vi "Process-Logging.vi"(9 "Wait on post-processing":refnum<k4>, 10 "Queues Cluster":T1, 11 "Data-gen queue":T2) -> (0 "error out":errorcluster)   [LabVIEW 2020]
uses:
  Logging/Typedefs/ROI File Generator Queue Ref.ctl
  Typedefs/Logging queue element.ctl
  Typedefs/Imaging Protocols enum.ctl
  Typedefs/Frame Size.ctl
  Typedefs/Acquired points count.ctl
  User Interface/Queue/Message Queue/Typedefs/All Message Queues.ctl
  User Interface/Queue/Message Queue/Typedefs/Message Cluster.ctl
  Global Variables/General Globals.vi
panel:
  out "Loop iterations":i32
  out "Number of trials closed":u32
  out "Loop period (ms)":u32
  # "TIME-CRITICAL MODULE"
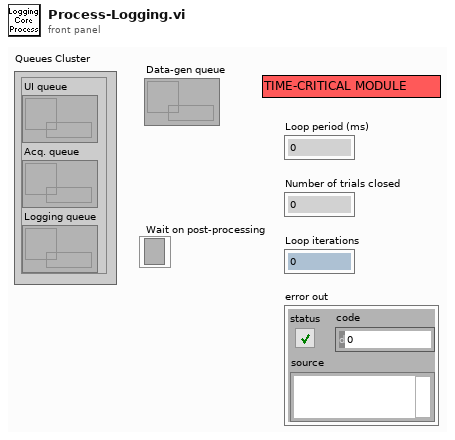
[diagram p1: front panel]
types:
  T1 = typedef "All Message Queues.ctl" = cluster{"UI queue":refnum<queue>, "Acq. queue":refnum<queue>, "Logging queue":refnum<queue>}
  T2 = typedef "ROI File Generator Queue Ref.ctl" = refnum<queue>
  T3 = cluster{"TDMS group name":string, "TDMS channel names array":string[]}
  T4 = typedef "Live graph data queue ref.ctl" = refnum<queue>
  T5 = typedef "Live imaging queue element.ctl" = cluster{"Red channel":T6, "Green channel":T6, "Ref Red channel":T6, "Ref Green channel":T6, "Mov cor":bool}
  T6 = typedef "IMAQ Image.ctl" = refnum<image>
  T7 = typedef "Logging queue element.ctl" = cluster{"Imaging Protocol":T8, "Number of Trials":u16, "Frame Size":T9, "# Averaged frames":u16, "Dwell time (us)":dbl, "Index of Z-plane":i32, "Timelapse?":bool, "Logging process is active":bool, "Speed logging enabled":bool, "tdms file ref":refnum<k34>, "path":path, "Trial Number":i32, "Expected # points acquired":bool, "Manually stopped":bool, "Last trial":bool, "Ch0 data":u32[], "Ch1 data":u32[], "Ref Data":u32[], "Ref Frame Time":u64[], "Image Time":u64[], "Continuous Time":u64[], "Ref X Length":u16, "Ref Y Length":u16, "# Ref Averaged frames":u16, "Ref Dwell time (us)":dbl, "Points acquired":T10, "HW Timings File":refnum<file>}
  T8 = typedef "Imaging Protocols enum.ctl" = enum16{"AOL Z-Stack", "Motor Z Stack", "Functional Acquisition", "Single Plane Acquisition", "Volume Acquisition", "Live Imaging", "Live Plane Imaging", "Live Volume Imaging"}
  T9 = typedef "Frame Size.ctl" = u16
  T10 = typedef "Acquired points count.ctl" = cluster{"Ch0 last trial":u64, "Ch1 last trial":u64, "All trials":u64}
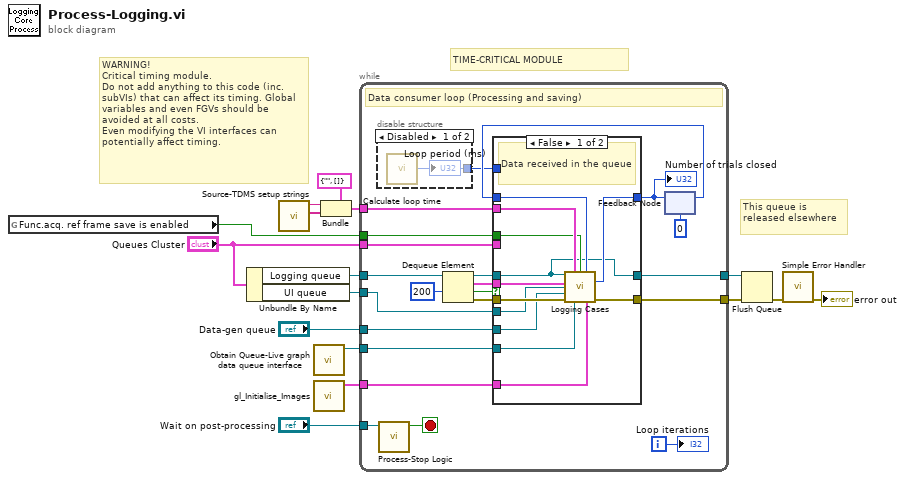
[diagram p0: block diagram]
diagram:
  # "WARNING!\nCritical timing module.\nDo not add anything to this code (inc. subVIs) that can affect its timing. Global variables and even FGVs should be avoided at all costs.\nEven modifying the VI interfaces can potentially affect timing."
  # "TIME-CRITICAL MODULE"
  # "This queue is released elsewhere"
  n1 = global read "General Globals.vi" "Func.acq. ref frame save is enabled"() -> (w2:bool)
  n2 = Unbundle By Name("Queues Cluster") -> ("Logging queue"=w4:refnum<queue>, "UI queue"=w1:refnum<queue>)
  n3 = call "Source-TDMS setup strings.vi"() -> ("Functional imaging TDMS channel names array"=w6:string[], "TDMS group name"=w7:string)  [unwired: 10 in]
  n4 = call "Obtain Queue-Live graph data queue interface.vi"() -> ("Live graphs queue"=w14:T4)  [unwired: 10 in, 1 out]
  n5 = call "gl_Initialise_Images.vi"() -> ("Live image refs"=w13:T5)  [unwired: 11 in]
  n6 = Bundle(cluster=T3 {"TDMS group name"="", "TDMS channel names array"=[]} ("Channel info"), "TDMS group name"=w7, "TDMS channel names array"=w6) -> (w5:T3)
  n7 = while {
    tunnel: [w35] -> w9
    tunnel: "Data-gen queue" -> [w33]
    tunnel: w13 -> [w31]
    tunnel: w14 -> [w29]
    tunnel: w4 -> [w34]
    tunnel: [w21] -> w10
    tunnel: "Wait on post-processing" -> [w22]
    tunnel: w5 -> [w24]
    tunnel: "Queues Cluster" -> [w20]
    tunnel: w2 -> [w19]
    tunnel: w1 -> [w18]
    i -> [w30]
    stop <- w23 stop-if-true
    # "Data consumer loop (Processing and saving)"
    n8 = disable-structure shown="Disabled" {
      disable-tunnel: [w39 _] -> w25
      frame Disabled {
        n9 = call <userlib>:"Calculate loop time.vi"() -> ("Loop time (ms)"=w39:u32)  [unwired: 11 in]
        "Loop period (ms)" <- w39
      }
      frame Enabled {
      }
    }
    n10 = call "Process-Stop Logic.vi"("Wait on post-processing"=w22) -> ("Abort logging"=w23:bool)  [unwired: 10 in]
    n11 = Dequeue Element(queue=w34, timeout in ms (-1)=200) -> (queue out=w17:refnum<queue>, element=w37:T7, timed out?=w28:bool, error out=w38:errorcluster)  [unwired: 1 in]
    n12 = feedback #1(u32 0 ("Number of files closed")) -> (w32:u32)
    n13 = case shown="False" w28 {
      tunnel: [w51 w54] -> w35
      tunnel: w38 -> [w50 w54]
      tunnel: w37 -> [w48 _]
      tunnel: w33 -> [w49 _]
      tunnel: [w43 w53] -> w27
      tunnel: w32 -> [w44 w53]
      tunnel: w31 -> [w46 _]
      tunnel: w29 -> [w47 _]
      tunnel: w17 -> [w41 w52]
      tunnel: w25 -> [_ _]
      tunnel: w24 -> [w45 _]
      tunnel: [w41 w52] -> w21
      tunnel: w20 -> [_ _]
      tunnel: w19 -> [w42 _]
      tunnel: w18 -> [w40 _]
      frame False {
        # "Data received in the queue"
        n14 = call "Logging Cases.vi"("Logging queue"=w41, "Channel info"=w45, "Enable ref saving during functional acq."=w42, "Number of files closed in"=w44, "Logging queue element in"=w48, "UI queue"=w40, "Data-gen queue"=w49, "error in"=w50, "Live graph data queue in"=w47, "Image array"=w46) -> ("Number of TDMS files closed"=w43:u32, "error out"=w51:errorcluster)  [unwired: 4 in]
      }
      frame True {
        # "Timed out (200ms). This case allows stopping the loop correctly."
      }
    }
    "Number of trials closed" <- w27
    n15 = feedback-in #1(w27) -> ()
    "Loop iterations" <- w30
  }
  n16 = Flush Queue(queue=w10, error in (no error)=w9) -> (error out=w11:errorcluster)  [unwired: 2 out]
  n17 = call <vilib>:"Simple Error Handler.vi"("error in (no error)"=w11) -> ("error out"=→"error out":errorcluster)  [unwired: 4 in, 4 out]
